vi "Joystick.vi"(8 "error in (no error)":errorcluster, 10 "Joystick":bool, 11 "Gantry In":refnum<k24>) -> (0 "error out":errorcluster, 3 "Gantry Out":refnum<k24>)   [LabVIEW 2020, in "A3200.lvclass"]
uses:
  A3200.lvclass
  Drivers/Aerotech A3200/Aerotech.lvlib
  C:/Program Files (x86)/Aerotech/A3200/LabVIEW/2010/Bin/Aerotech.A3200.dll
  Program Files (x86)/Aerotech/A3200/LabVIEW/2010/Bin/Aerotech.A3200.dll
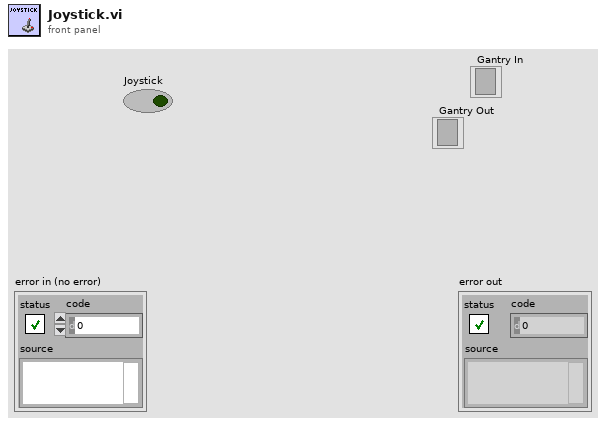
[diagram p1: front panel]
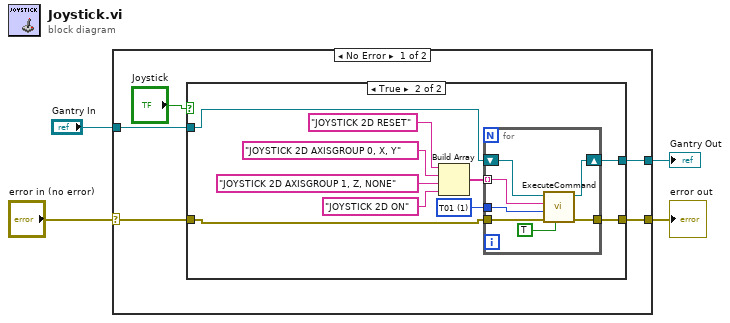
[diagram p0: block diagram]
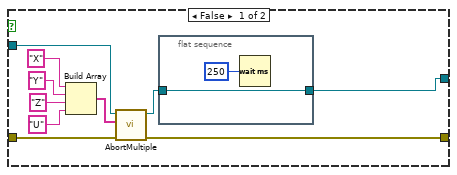
[diagram p2: hidden frame]
diagram:
  n1 = case shown="No Error" "error in (no error)" {
    selector: "error in (no error)" -> [w6 w40]
    tunnel: [w5 w40] -> w3
    tunnel: "Gantry In" -> [w8 w39]
    tunnel: [w7 w39] -> w1
    frame No Error {
      n2 = case shown="True" "Joystick" {
        tunnel: [w13 w24] -> w7
        tunnel: w8 -> [w12 w25]
        tunnel: w6 -> [w10 w23]
        tunnel: [w11 w22] -> w5
        frame False {
          n3 = Build Array("X" ("axis name"), "Y", "Z", "U") -> (w15:string[])
          n4 = call "AbortMultiple.vi"("error in (no error)"=w10, "axis names"=w15, "controller in"=w12) -> ("error out"=w11:errorcluster, "controller out"=w14:refnum<k24>)  [unwired: 7 in]
          n5 = flat-sequence {
            tunnel: w14 -> [w21]
            tunnel: [w21] -> w13
            frame #0 {
              n6 = Wait (ms)(milliseconds to wait=u32 250) -> ()  [unwired: 1 out]
            }
          }
        }
        frame True {
          w27 = 1 items=["TLibrary", "T01", "T02", "T03", "T04", "T05", "T06", "T07", "T08", "T09", "T10", "T11", "T12", "T13", "T14", "T15", "T16", "T17", "T18", "T19", "T20", "T21", "T22", "T23", "T24", "T25", "T26", "T27", "T28", "T29", "T30", "T31"] ("taskId")
          n7 = Build Array("JOYSTICK 2D RESET", "JOYSTICK 2D AXISGROUP 0, X, Y", "JOYSTICK 2D AXISGROUP 1, Z, NONE", "JOYSTICK 2D ON") -> (w28:string[])
          n8 = for {
            tunnel: w28 -> [w38] mode=indexing
            tunnel: w27 -> [w37]
            shift-right: [w34] -> w24
            shift-left: w25 -> [w35]
            tunnel: w23 -> [w33]
            tunnel: [w32] -> w22
            n9 = call "ExecuteCommand.vi"("return immediately"=TRUE, "error in (no error)"=w33, "taskId"=w37, "Command Code"=w38, "controller in"=w35) -> ("error out"=w32:errorcluster, "controller out"=w34:refnum<k24>)  [unwired: 4 in, 1 out]
          }
        }
      }
    }
    frame Error {
    }
  }
  "error out" <- w3
  "Gantry Out" <- w1
